vi "Get Data.vi"(8 "error in (no error)":errorcluster, 11 "Tree Data File in":refnum<class "Tree Data File.lvclass">) -> (0 "error out":errorcluster, 3 "Tree Data File out":refnum<class "Tree Data File.lvclass">)   [LabVIEW 2024, in "Tree Data File.lvclass"]
uses:
  Tree Data File.lvclass
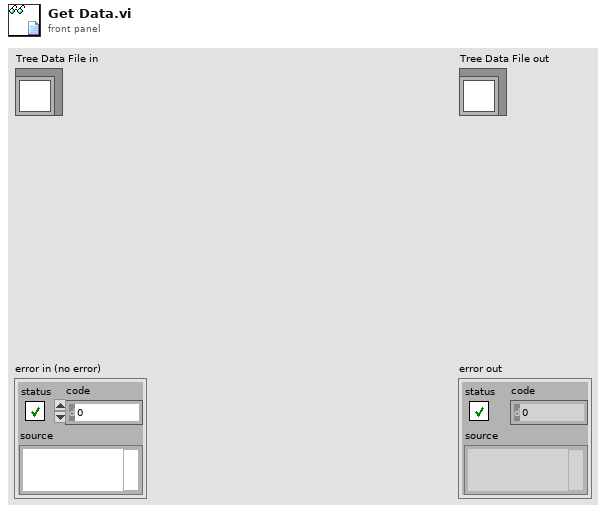
[diagram p1: front panel]
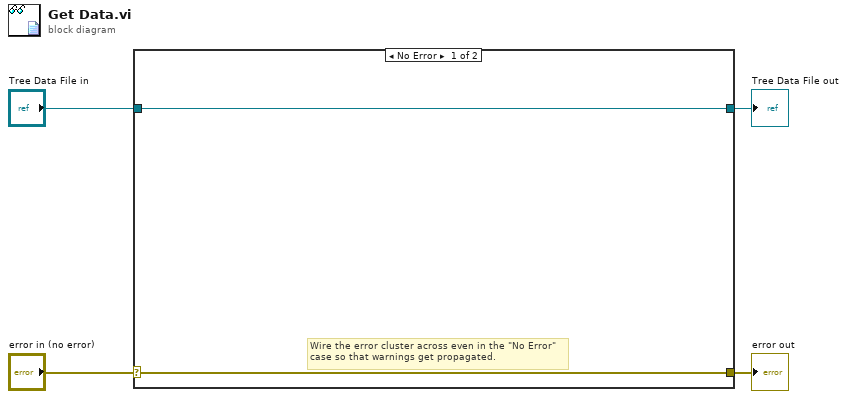
[diagram p0: block diagram]
diagram:
  n1 = case shown="No Error" "error in (no error)" {
    selector: "error in (no error)" -> [w6 w8]
    tunnel: [w6 w8] -> w3
    tunnel: [w5 w7] -> w1
    tunnel: "Tree Data File in" -> [w5 w7]
    frame No Error {
      # "Wire the error cluster across even in the \"No Error\"\ncase so that warnings get propagated."
    }
    frame Error {
    }
  }
  "error out" <- w3
  "Tree Data File out" <- w1
